vi "TS Acq Stop.vi"(8 "error in":errorcluster, 11 "DeepU Test Stand in":refnum<class "DeepU Test Stand.lvclass">) -> (0 "error out":errorcluster, 3 "DeepU Test Stand out":refnum<class "DeepU Test Stand.lvclass">)   [LabVIEW 2019, in "Test Stands.lvlib" / "DeepU Test Stand.lvclass"]
uses:
  DeepU Test Stand.lvclass
  DeepU Test Stand.lvclass/DeepU Test Stand.ctl
  <vilib>/DAQmx/write.llb/DAQmx Write (Digital Bool 1Line 1Point).vi
  <vilib>/DAQmx/miscellaneous.llb/DAQmx Fill In Error Info.vi
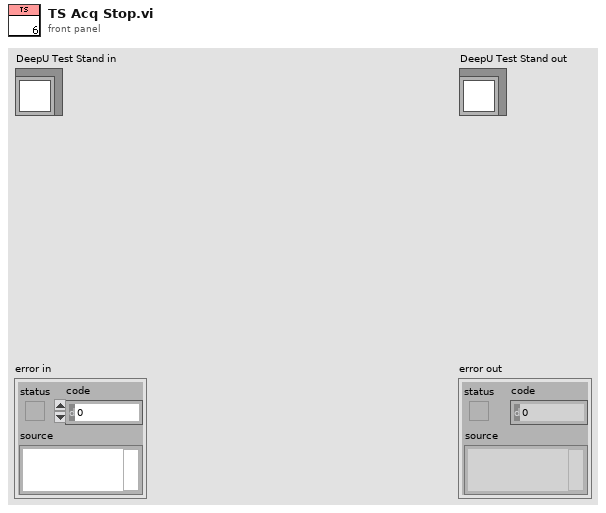
[diagram p1: front panel]
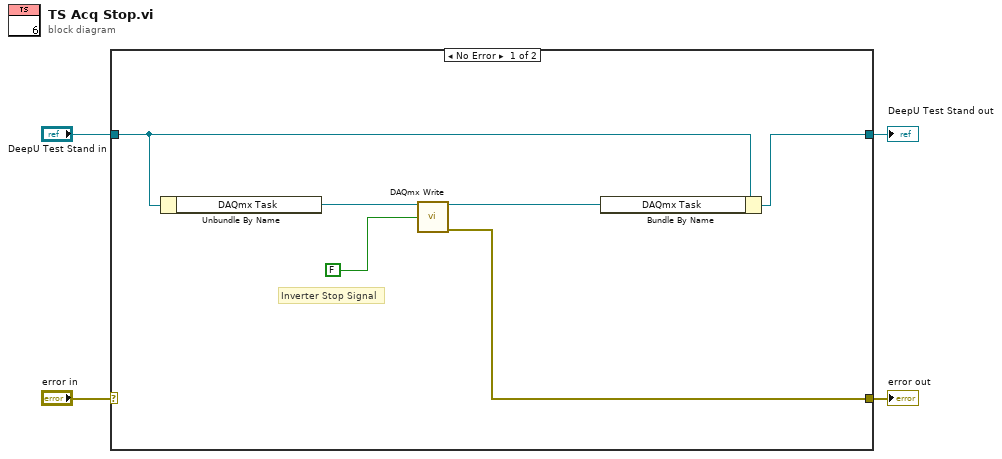
[diagram p0: block diagram]
diagram:
  n1 = case shown="No Error" "error in" {
    selector: "error in" -> [_ w12]
    tunnel: [w6 w12] -> w1
    tunnel: [w9 w11] -> w3
    tunnel: "DeepU Test Stand in" -> [w10 w11]
    frame No Error {
      # "Inverter Stop Signal"
      n2 = Unbundle By Name(w10) -> ("DAQmx Task"=w8:refnum<k21>)
      n3 = call-poly <vilib>:"DAQmx Write.vi"("task/channels in"=w8, "data"=FALSE) -> ("task out"=w7:refnum<k21>, "error out"=w6:errorcluster)  [unwired: 11 in, 1 out]
      n4 = Bundle By Name(cluster=w10, "DAQmx Task"=w7) -> (w9:refnum<class "DeepU Test Stand.lvclass">)
    }
    frame Error {
    }
  }
  "error out" <- w1
  "DeepU Test Stand out" <- w3
